vi "String_match (SubVI).vi"(0 "channel id":string, 3 "input string":string, 4 "Boolean in":bool, 5 "error in":errorcluster) -> (10 "match ?":i32, 14 "output string":string, 17 "match substring":string, 18 "Boolean out":bool, 19 "error out":errorcluster)   [LabVIEW 2013]
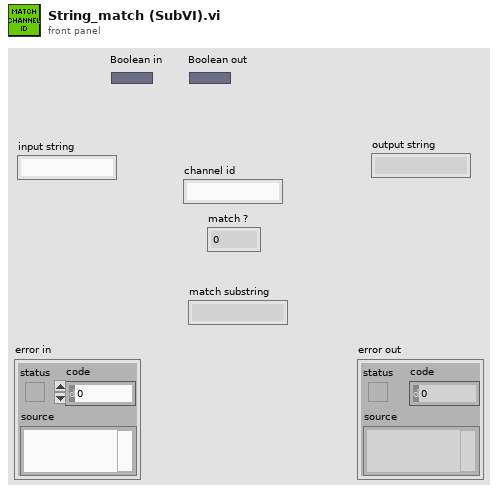
[diagram p1: front panel]
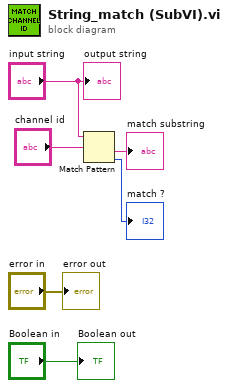
[diagram p0: block diagram]
diagram:
  n1 = Match Pattern(string="input string", regular expression="channel id") -> (after substring=→"match substring":string, offset past match=→"match ?":i32)  [unwired: 3 out]
  "output string" <- "input string"
  "error out" <- "error in"
  "Boolean out" <- "Boolean in"
